vi "Setup UI.vi"(8 "error in (no error)":errorcluster, 10 "Set UI to input? (F)":bool, 11 "Magna Voltage Scan in":refnum<class "Magna Voltage Scan.lvclass">) -> (0 "error out":errorcluster, 3 "Magna Voltage Scan out":refnum<class "Magna Voltage Scan.lvclass">)   [LabVIEW 2015, in "Magna Voltage Scan.lvclass"]
doc: "Scanner::Setup is a constructor that has no parameters and faces the user. The Factory calls this VI to let the user configure this Scanner. It is dynamically dispatched in order to let the user choose the type as well as the options of the scanner."
uses:
  Magna Voltage Scan.lvclass
  Magna Voltage Scan.lvclass/Magna Voltage Scan.ctl
  Instruments/Magna-Power Power Supply/Magna Power.lvclass
  Instruments/Magna-Power Power Supply/Magna Power Constants.vi
  <vilib>/gmath/NI_Gmath.lvlib
panel:
  in  "Voltage Limit":dbl=2255.0
  out "Positive?":bool
  in  "Go to first\ncoordinate (roughly)":bool
  in  "Sweep rate (T/s)":dbl
  # "Magna Voltage Setup"
  # "A positive field corresponds to a north pole located on the right when looking straight on at magnet"
  # "Usually set to 2255 V"
  # "(Button will stay\ngreen when pressed)"
  # "Max field ~ 1.36 T\nAlways enter positive field values.\n\nMay behave strangely for fields below 0.05 T,\nbut a \"Return to\" value of 0 is valid."
  # "If you want to do multiple scans, you must check the \"Return to\" box and enter the first point of your scan."
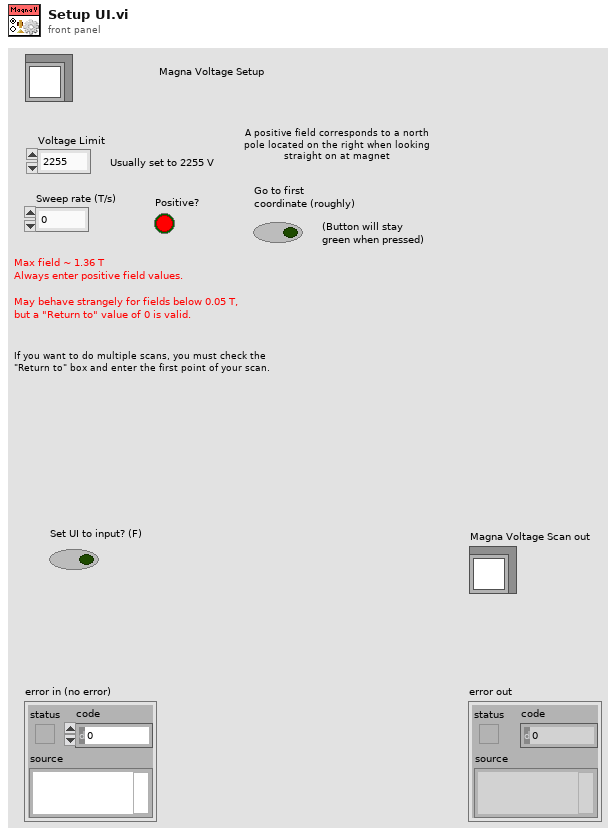
[diagram p1: front panel]
types:
  T1 = typedef "Scanner.lvclass/Range.ctl" = cluster{"xi":dbl, "xf":dbl, "dx":dbl, "Return to...?":bool, "Return to":dbl}
  T2 = cluster{"Magna Current":dbl[], "Magnetic Field":dbl[], "Fluke Voltage":dbl[]}
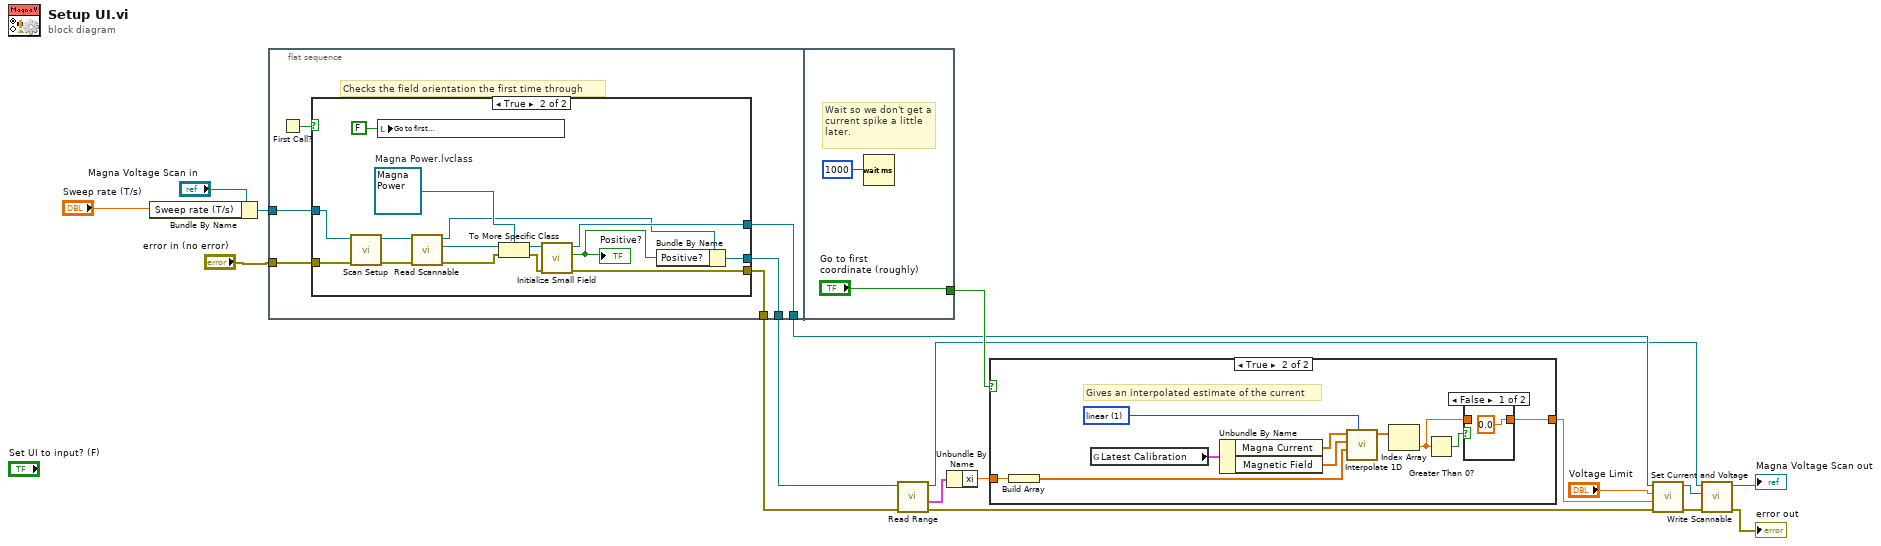
[diagram p0: block diagram]
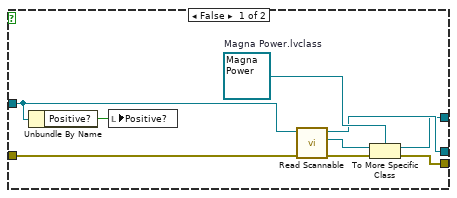
[diagram p2: hidden frame]
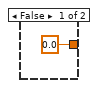
[diagram p3: hidden frame]
diagram:
  n1 = Bundle By Name(cluster="Magna Voltage Scan in", "Sweep rate (T/s)"="Sweep rate (T/s)") -> (w13:refnum<class "Magna Voltage Scan.lvclass">)
  n2 = flat-sequence {
    tunnel: "error in (no error)" -> [w23]
    tunnel: w13 -> [w22]
    tunnel: [w21] -> w8
    tunnel: [w20] -> w10
    tunnel: [w19] -> w12
    tunnel: ["Go to first\ncoordinate (roughly)"] -> w15
    frame #0 {
      # "Checks the field orientation the first time through"
      n3 = First Call?() -> (First Call?: T/F=w24:bool)
      n4 = case shown="True" w24 {
        tunnel: w22 -> [w26 w44]
        tunnel: w23 -> [w29 w43]
        tunnel: [w32 w35] -> w21
        tunnel: [w28 w39] -> w20
        tunnel: [w27 w38] -> w19
        frame False {
          w33 = refnum<class "Magna Power.lvclass"> refnum  # Magna Power.lvclass
          n5 = Unbundle By Name(w26) -> ("Positive?"=w25:bool)
          n6 = local write "Positive?"(w25) -> ()
          n7 = call-dynamic "Read Scannable.vi"("error in (no error)"=w29, "Scanner.lvclass in"=w26) -> ("error out"=w31:errorcluster, "Scannable.lvclass"=w30:refnum<class "Scannable.lvclass">, "Scanner.lvclass out"=w32:refnum<class "Magna Voltage Scan.lvclass">)  [unwired: 7 in]
          n8 = To More Specific Class(target class=w33, reference=w30, error in=w31) -> (specific class reference=w27:refnum<class "Magna Power.lvclass">, error out=w28:errorcluster)
        }
        frame True {
          w46 = refnum<class "Magna Power.lvclass"> refnum  # Magna Power.lvclass
          n9 = call-dynamic "Scan Setup.vi"("error in (no error)"=w43, "Magna Voltage Scan in"=w44) -> ("error out"=w42:errorcluster, "Magna Voltage Scan out"=w37:refnum<class "Magna Voltage Scan.lvclass">)  [unwired: 8 in]
          n10 = local write "Go to first\ncoordinate (roughly)"(FALSE ("Go to first coordinate (roughly)")) -> ()
          n11 = call-dynamic "Read Scannable.vi"("error in (no error)"=w42, "Scanner.lvclass in"=w37) -> ("error out"=w47:errorcluster, "Scannable.lvclass"=w45:refnum<class "Scannable.lvclass">, "Scanner.lvclass out"=w36:refnum<class "Magna Voltage Scan.lvclass">)  [unwired: 7 in]
          n12 = To More Specific Class(target class=w46, reference=w45, error in=w47) -> (specific class reference=w40:refnum<class "Magna Power.lvclass">, error out=w41:errorcluster)
          n13 = call "Initialize Small Field.vi"("error in (no error)"=w41, "Magna Power in"=w40) -> ("error out"=w39:errorcluster, "Positive?"=w34:bool, "Magna Power out"=w38:refnum<class "Magna Power.lvclass">)  [unwired: 7 in]
          "Positive?" <- w34
          n14 = Bundle By Name(cluster=w36, "Positive?"=w34) -> (w35:refnum<class "Magna Voltage Scan.lvclass">)
        }
      }
    }
    frame #1 {
      # "Wait so we don't get a current spike a little later."
      n15 = Wait (ms)(milliseconds to wait=u32 1000) -> ()  [unwired: 1 out]
    }
  }
  n16 = call-dynamic "Read Range.vi"("error in (no error)"=w10, "Scanner.lvclass in"=w8) -> ("error out"=w9:errorcluster, "Range"=w11:T1, "Scanner.lvclass out"=w7:refnum<class "Magna Voltage Scan.lvclass">)  [unwired: 4 in, 3 out]
  n17 = Unbundle By Name(w11) -> ("xi"=w6:dbl)
  n18 = case shown="True" w15 {
    tunnel: [0.0 ("Current Limit") w53] -> w14
    tunnel: w6 -> [_ w52]
    frame False {
    }
    frame True {
      w60 = 1 items=["nearest", "linear", "spline", "cubic Hermite", "Lagrange"] ("method")
      # "Gives an interpolated estimate of the current"
      n19 = Build Array(w52) -> (w59:dbl[])
      n20 = global read "Magna Power Constants.vi" "Latest Calibration"() -> (w61:T2)
      n21 = Unbundle By Name(w61) -> ("Magna Current"=w56:dbl[], "Magnetic Field"=w57:dbl[])
      n22 = call <vilib>:"Interpolate 1D.vi"("method"=w60, "xi"=w59, "X"=w57, "Y"=w56) -> ("yi"=w58:dbl[])  [unwired: 5 in, 2 out]
      n23 = Index Array(array=w58) -> (element=w54:dbl)  [unwired: 1 in]
      n24 = Greater Than 0?(x=w54) -> (x > 0?=w55:bool)
      n25 = case shown="False" w55 {
        tunnel: [0.0 ("Numeric") w63] -> w53
        tunnel: w54 -> [_ w63]
        frame False {
        }
        frame True {
        }
      }
    }
  }
  n26 = call "Set Current and Voltage.vi"("error in (no error)"=w9, "Current Limit"=w14, "Voltage Limit"="Voltage Limit", "Magna Power in"=w12) -> ("error out"=w18:errorcluster, "Magna Power out"=w17:refnum<class "Magna Power.lvclass">)  [unwired: 6 in]
  n27 = call-dynamic "Write Scannable.vi"("error in (no error)"=w18, "Scannable.lvclass"=w17, "Scanner.lvclass in"=w7) -> ("error out"=→"error out":errorcluster, "Scanner.lvclass out"=→"Magna Voltage Scan out":refnum<class "Magna Voltage Scan.lvclass">)  [unwired: 7 in]
